vi "Image_Pro_controls_to_string.vi"(6 "Camera":string, 8 "ROI to crop (pixels)":T1={"Xmax"=2147483647, "Ymax"=2147483647, "Xmin"=0, "Ymin"=0}, 9 "Txy range (pixels)":T2={"Tx max (pix)"=2147483647, "Tx min (pix)"=-2147483648, "Ty max (pix)"=2147483647, "Ty min (pix)"=-2147483648}, 10 "Theta range (deg)":T4={"theta max (deg)"=180.0, "theta min (deg)"=-180.0} {"theta min (deg)" min=-360.0 max=360.0; "theta max (deg)" min=-360.0 max=360.0}, 11 "Controls":T3={"Auto ROI (for rot.)"=FALSE, "Apply scaling"=FALSE, "Apply rotation"=TRUE, "Apply Tx"=TRUE, "Apply Ty"=TRUE, "Keep proc. img"=FALSE}) -> (1 "Setup String":string)   [LabVIEW 2015]
uses:
  Typedefs/Theta range.ctl
  Typedefs/Top level controls.ctl
  Typedefs/Txy range.ctl
  Typedefs/ROI bounds.ctl
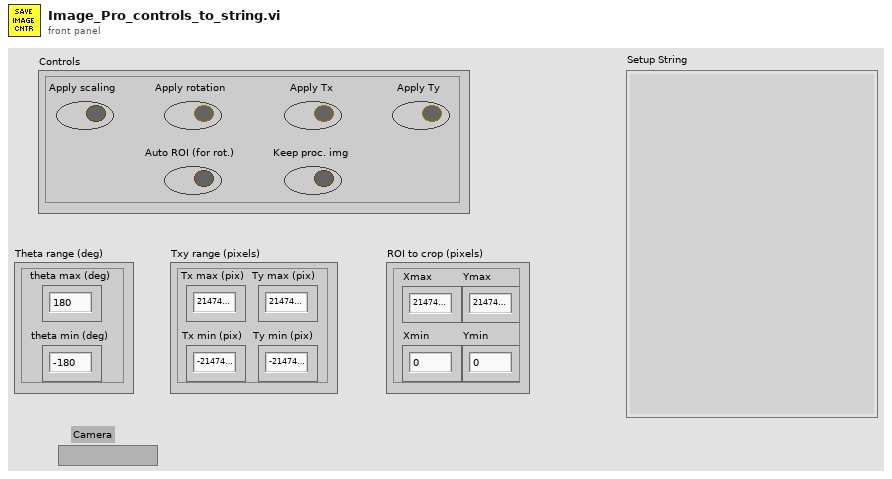
[diagram p1: front panel]
types:
  T1 = typedef "ROI bounds.ctl" = cluster{"Xmax":i32, "Ymax":i32, "Xmin":i32, "Ymin":i32}
  T2 = typedef "Txy range.ctl" = cluster{"Tx max (pix)":i32, "Tx min (pix)":i32, "Ty max (pix)":i32, "Ty min (pix)":i32}
  T3 = typedef "Top level controls.ctl" = cluster{"Auto ROI (for rot.)":bool, "Apply scaling":bool, "Apply rotation":bool, "Apply Tx":bool, "Apply Ty":bool, "Keep proc. img":bool}
  T4 = typedef "Theta range.ctl" = cluster{"theta max (deg)":dbl, "theta min (deg)":dbl}
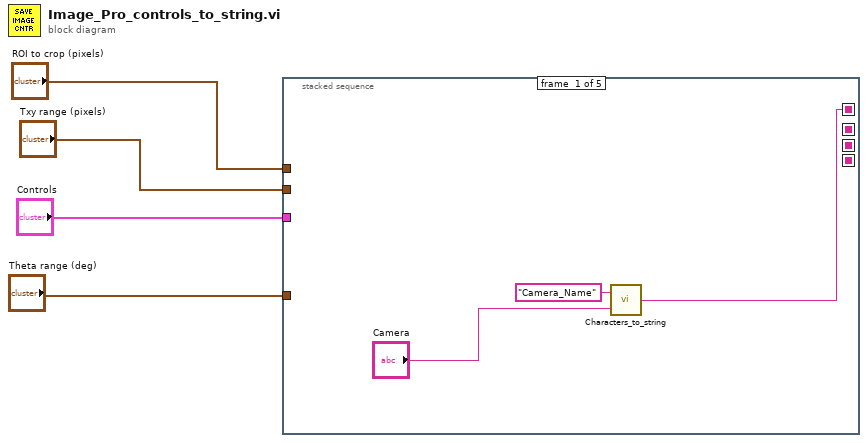
[diagram p0: block diagram]
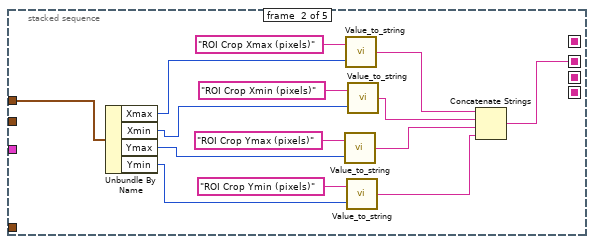
[diagram p2: hidden frame]
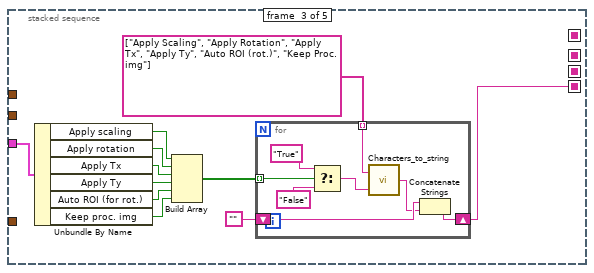
[diagram p3: hidden frame]
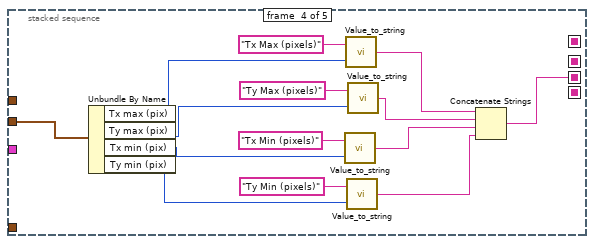
[diagram p4: hidden frame]
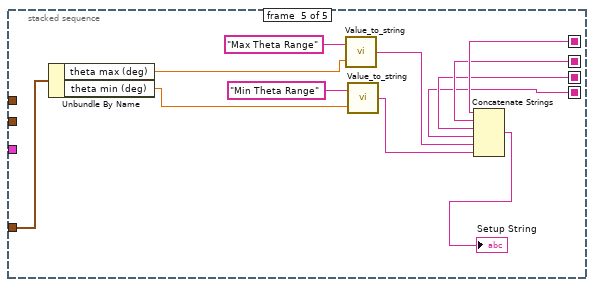
[diagram p5: hidden frame]
diagram:
  n1 = stacked-sequence {
    seq-local: [w5 _ _ _ _] -> [_ _ _ _ w60]
    seq-local: [_ w8 _ _ _] -> [_ _ _ _ w59]
    seq-local: [_ _ _ w41 _] -> [_ _ _ _ w58]
    seq-local: [_ _ w23 _ _] -> [_ _ _ _ w56]
    tunnel: "ROI to crop (pixels)" -> [_ w18 _ _ _]
    tunnel: "Theta range (deg)" -> [_ _ _ _ w61]
    tunnel: "Txy range (pixels)" -> [_ _ _ w42 _]
    tunnel: "Controls" -> [_ _ w22 _ _]
    frame #0 {
      n2 = call "Characters_to_string.vi"("Characters to write"="Camera", "Label for characters"="Camera_Name") -> ("Output string"=w5:string)
    }
    frame #1 {
      n3 = Unbundle By Name(w18) -> ("Xmax"=w14:i32, "Xmin"=w15:i32, "Ymax"=w16:i32, "Ymin"=w17:i32)
      n4 = call "Value_to_string.vi"("Value"=w16, "Label for value"="ROI Crop Ymax (pixels)" ("Label for characters")) -> ("Output string"=w11:string)  [unwired: 1 in]
      n5 = call "Value_to_string.vi"("Value"=w14, "Label for value"="ROI Crop Xmax (pixels)" ("Label for characters")) -> ("Output string"=w13:string)  [unwired: 1 in]
      n6 = call "Value_to_string.vi"("Value"=w17, "Label for value"="ROI Crop Ymin (pixels)" ("Label for characters")) -> ("Output string"=w10:string)  [unwired: 1 in]
      n7 = call "Value_to_string.vi"("Value"=w15, "Label for value"="ROI Crop Xmin (pixels)" ("Label for characters")) -> ("Output string"=w12:string)  [unwired: 1 in]
      n8 = Concatenate Strings(w13, w12, w11, w10) -> (w8:string)
    }
    frame #2 {
      n9 = Unbundle By Name(w22) -> ("Apply scaling"=w32:bool, "Apply rotation"=w31:bool, "Apply Tx"=w30:bool, "Apply Ty"=w29:bool, "Auto ROI (for rot.)"=w28:bool, "Keep proc. img"=w27:bool)
      n10 = Build Array(w32, w31, w30, w29, w28, w27) -> (w26:bool[])
      n11 = for {
        tunnel: w26 -> [w40] mode=indexing
        tunnel: string[] ["Apply Scaling", "Apply Rotation", "Apply Tx", "Apply Ty", "Auto ROI (rot.)", "Keep Proc. img"] -> [w36] mode=indexing
        shift-right: [w35] -> w23
        shift-left: "" -> [w34]
        n12 = Select(t="True", s=w40, f="False") -> (s? t:f=w37:string)
        n13 = call "Characters_to_string.vi"("Characters to write"=w37, "Label for characters"=w36) -> ("Output string"=w33:string)
        n14 = Concatenate Strings(w34, w33) -> (w35:string)
      }
    }
    frame #3 {
      n15 = Unbundle By Name(w42) -> ("Tx max (pix)"=w48:i32, "Ty max (pix)"=w49:i32, "Tx min (pix)"=w50:i32, "Ty min (pix)"=w51:i32)
      n16 = call "Value_to_string.vi"("Value"=w50, "Label for value"="Tx Min (pixels)" ("Label for characters")) -> ("Output string"=w45:string)  [unwired: 1 in]
      n17 = call "Value_to_string.vi"("Value"=w48, "Label for value"="Tx Max (pixels)" ("Label for characters")) -> ("Output string"=w47:string)  [unwired: 1 in]
      n18 = call "Value_to_string.vi"("Value"=w51, "Label for value"="Ty Min (pixels)" ("Label for characters")) -> ("Output string"=w44:string)  [unwired: 1 in]
      n19 = call "Value_to_string.vi"("Value"=w49, "Label for value"="Ty Max (pixels)" ("Label for characters")) -> ("Output string"=w46:string)  [unwired: 1 in]
      n20 = Concatenate Strings(w47, w46, w45, w44) -> (w41:string)
    }
    frame #4 {
      n21 = Unbundle By Name(w61) -> ("theta max (deg)"=w63:dbl, "theta min (deg)"=w64:dbl)
      n22 = call "Value_to_string.vi"("Value"=w63, "Label for value"="Max Theta Range" ("Label for characters")) -> ("Output string"=w57:string)  [unwired: 1 in]
      n23 = call "Value_to_string.vi"("Value"=w64, "Label for value"="Min Theta Range" ("Label for characters")) -> ("Output string"=w62:string)  [unwired: 1 in]
      n24 = Concatenate Strings(w60, w59, w58, w56, w57, w62) -> (→"Setup String":string)
    }
  }
